vi "NI-USB6343.vi"() -> ()   [LabVIEW 2020]
uses:
  LabVIEW 2020 Toolkits/VI Server Toolkit/VI Server Toolkit LV2013.lvlib
  LabVIEW 2020 Toolkits/toolkits_lv2020_32bit/Synchronization.llb/SynchRefs_SetGet.ctl
  LabVIEW 2020 Toolkits/VI Server Toolkit/VI Server Libraries/VI Server_GetControl.llb/VI Server_STR_Get.vi
  LabVIEW 2020 Toolkits/VI Server Toolkit/VI Server Libraries/VI Server_Set Controls.llb/Set STR Control.vi
  LabVIEW 2020 Toolkits/VI Server Toolkit/VI Server Libraries/VI Server_GetControl.llb/VI Server_DAQmx_Device_Get.vi
panel:
  in  "LastAction.AddToSecuence":bool
  out "System.Message":string caption="System Message"
  in  "Help":bool
  in  "FP.Hide":bool caption="FrontPanel.Hide"
  in  "EXIT":bool
  in  "Tab.Main":T1(tab)
  out "AI.ActualSampleRate":dbl=1000.0 caption="Actual Sample Rate" format="%0.2f"
  out "AI.WaveformGraph":waveform(dbl)(graph) caption="Waveform Graph"
  out "AI.Averaged.Mesurement":dbl caption="Averaged Mesurement" format="%0.4f V"
  in  "AI.Measure":bool caption="AI:Measure"
  in  "AI.Number.Of.Samples":i32=100 caption="Number Of Samples"
  in  "AI.SampleRate":dbl=1000.0 caption="Sample Rate" format="%0.0f Hz"
  in  "AI.MinInputLimit":dbl caption="Min Input Limit" min=-10.0 max=10.0 format="%0.3f V"
  in  "AI.MaxInputLimit":dbl caption="Max Input Limit" min=-10.0 max=10.0 format="%0.3f V"
  in  "AI.TerminalConfiguration":u16(ring)=65535 caption="Terminal Configuration" items=["default"=65535, "RSE"=10083, "NRSE"=10078, "Differential"=10106, "Pseudodifferential"=12529]
  in  "AI.Sample.Mode":u16(ring)=12522 caption="Sample Mode" items=["Finite Samples"=10178, "Continuous Samples"=10123]
  in  "AI.Physical.Channel":tag="Dev1/ai0" caption="Physical Channel"
  in  "AO.GenerationMode":u16(ring) caption="Generation Mode" items=["Voltage DC", "Voltage Sine Wave Generation", "Voltage Triangle Wave Generation", "Voltage Square Wave Generation", "Voltage Sawtooth Wave Generation"]
  in  "AO.Physical.Channel":tag="Dev1/ai0" caption="Physical Channel"
  in  "AO.Update":bool
  in  "AO.Output":bool caption="AO:Output"
  out "AO.WaveformGraph":waveform(dbl)(graph) caption="Waveform Graph"
  in  "AO.SampleMode":u16(ring) caption="Sample Mode" items=["Finite Samples"=10178, "Continious Samples"=10123, "Hardware Timed Single Point"=12522]
  in  "AO.NumberOfSamples":i32=1000 caption="Number Of Samples" min=2
  in  "AO.SampleRate":dbl=1000.0 caption="Sample Rate" format="%0.1f Hz"
  in  "AO.Sample.Clock.Source":tag="OnboardClock" caption="Sample Clock Source"
  out "AO.ActualSampleRate":dbl=1000.0 caption="Actual Sample Rate" format="%0.2f"
  in  "AO.OutputVoltage":dbl(slide) caption="Amplitude" min=-10.0 max=10.0 scale=-10.0..9.0 scale format="%0.3f V"
  in  "AO.SinewaveFrequency":dbl=10.0 caption="Sinewave Frequency" format="%0.2p Hz"
  in  "AO.MaxVoltage":dbl=5.0 caption="Max Voltage" format="%0.3f V"
  in  "AO.MinVoltage":dbl=-5.0 caption="Min Voltage" format="%0.3f V"
  in  "DO.Port.Mask.Apply":bool caption="DO:Port.Mask.Apply"
  in  "DO.Port.Lines.31:24.Mask":u8 caption="Port&Lines 31:24" format="%08b"
  in  "DO.Port.Lines.23:16.Mask":u8 caption="Port&Lines 23:16" format="%08b"
  in  "DO.Port.Lines.15:8.Mask":u8 caption="Port&Lines 15:8" format="%08b"
  in  "DO.Port.Lines.7:0.Mask":u8 caption="Port&Lines 7:0" format="%08b"
  out "DO.Port.State.Verify":bool caption="Verified"
  out "DO.Line.State.Verify":bool caption="Verified"
  in  "DO.Line.State":bool caption="State"
  in  "DO.Line":tag="Dev1/port0/line0:7" caption="Line"
  in  "DO.Line.Update":bool caption="Update:"
  in  "DO.Port.Update":bool caption="DO:Port.Update"
  in  "DO.Port.Lines.31:24":u8 caption="Port&Lines 31:24" format="%08b"
  in  "DO.Port.Lines.23:16":u8 caption="Port&Lines 23:16" format="%08b"
  in  "DO.Port.Lines.15:8":u8 caption="Port&Lines 15:8" format="%08b"
  in  "DO.Port.Lines.7:0":u8 caption="Port&Lines 7:0" format="%08b"
  in  "DO.Port":tag="Dev1/port0/line0:7" caption="Port"
  out "DI.Line.State":bool caption="State"
  in  "DI.Port.Update":bool caption="DI:Port.Update"
  out "DI.Port.Lines.24:31":u8 caption="Port&Lines 31:24" format="%08b"
  out "DI.Port.Lines.16:23":u8 caption="Port&Lines 23:16" format="%08b"
  out "DI.Port.Lines.8:15":u8 caption="Port&Lines 15:8" format="%.0b"
  out "DI.Port.Lines.0:7":u8 caption="Port&Lines 7:0" format="%.0b"
  in  "DI.Port":tag="Dev1/port0/line0:7" caption="Port"
  in  "DI.Line":tag="Dev1/port0/line0:7" caption="Line"
  in  "DI.Line.Update":bool caption="Update:"
  out "ctr3.Out.Duty Cycle.Actual":dbl caption="Ctr3: Duty Cycle Actual" format="%.2f"
  out "ctr3.Out.Frequency.Actual":dbl caption="Ctr3: Frequency Actual" format="%0.3f Hz"
  out "ctr2.Out.Duty Cycle.Actual":dbl caption="Ctr2: Duty Cycle Actual" format="%.2f"
  out "ctr2.Out.Frequency.Actual":dbl caption="Ctr2: Frequency Actual" format="%0.3f Hz"
  out "ctr1.Out.Duty Cycle.Actual":dbl caption="Ctr1: Duty Cycle Actual" format="%.2f"
  out "ctr1.Out.Frequency.Actual":dbl caption="Ctr1: Frequency Actual" format="%0.3f Hz"
  out "ctr0.Out.Duty Cycle.Actual":dbl caption="Ctr0: Duty Cycle Actual" format="%.2f"
  out "ctr0.Out.Frequency.Actual":dbl caption="Ctr0: Frequency Actual" format="%0.3f Hz"
  in  "Cntr.Out.NumberOfPulses":i32=1000 caption="Number Of Pulses" min=1
  in  "Cntr.Out.Start":bool
  in  "Cntr.Out.Sample.Mode":u16(ring)=10123 caption="Sample Mode" items=["Finite Samples"=10178, "Continuous Samples"=10123, "Hardware Timed Single Point"=12522]
  in  "Cntr.Out.Duty.Cycle":dbl=0.5 caption="Duty Cycle" format="%.2f %"
  in  "Cntr.Out.Frequency":dbl=1.0 caption="Frequency" format="%0.3f Hz"
  in  "Cntr.Out.Output.Terminal":tag="/Dev1/PFI12" caption="Output Terminal"
  in  "Cntr.Out.Channel":tag="Dev1/ctr0" caption="Channel"
  out "ctr3.In.Count":u32 caption="Count.3:"
  out "ctr2.In.Count":u32 caption="Count.2:"
  out "ctr1.In.Count":u32 caption="Count.1:"
  out "ctr0.In.Count":u32 caption="Count.0:"
  in  "Cntr.In.Start":bool
  in  "Cntr.In.IntegrationTime":u32=10 format="%.0f msec"
  in  "Cntr.In.Sample.Clock.Source":tag="PFI0" caption="Sample Clock Source"
  in  "Cntr.In.ActiveEdge":u16(ring)=10280 caption="Active Edge" items=["Rising"=10280, "Falling"=10171]
  in  "Cntr.In.Input.Terminal":tag="PFI8" caption="Input.Terminal"
  in  "Cntr.In.Channel":tag="Dev1/port0/line0:7" caption="Channel Name"
  in  "TestCase.Execute.All":bool
  in  "TestCase.Execute.Selected":bool
  out "TestCase.SAVE.Success":bool
  in  "TestCase.SAVE":bool
  in  "SequenceFile.Open":bool
  in  "SequenceFile":path caption="Secuence File"
  in  "TestCase.Execute.Step.Pause":bool
  in  "TestCase.Execute.Steps":u16(ring) caption="Test Case: Pause After Step" items=["1", "2", "3", "4"]
  in  "TestCase.Execute.ABORT":bool
  in  "TestCase.Execute.Next":bool
  in  "TestCase.Execute.Pause":bool
  out "TestCase.ExecutionTime":dbl caption="Execution Time:" format="%0.3f sec"
  in  "TestCase.Execution.StepTime":u32 caption="Seq. Execution: Step Time" format="%d msec"
  in  "TestCaseConfiguration":i32[](listbox) caption="Test Case Configuration"
  in  "TestCase.StepDescription":string caption="Step Description:"
  in  "ProductType":string="USB-6343 (BNC)" caption="Product Type"
  in  "VI.WindowsTitle":string caption="Windows Title"
  in  "DAQmx.Device":tag caption="DAQmx: Device"
  in  "Cont.Measurements.CycleTime":u32 caption="Continius Measurements:\nCycleTime"
  in  "UDP.Test.String2.Send":bool
  in  "UDP.Test.String2":string caption="UDP: Test String 2"
  in  "UDP.Port.BC":u16=58433 caption="UDP: Port.BC"
  in  "UDP.Port.RT":u16=58432 caption="UDP: Port.RT"
  in  "UDP.LocalPort":u16=58434 caption="UDP: Local Port"
  in  "UDP.IP.Address":string="234.5.6.7" caption="UDP: IP Address"
  in  "UDP.Test.String1.Send":bool
  in  "UDP.Test.String1":string caption="UDP: Test String 1"
  in  "UDP.Responce.String.Monitor":bool
  out "UDP.ExecEng.Message.String":string caption="UDP: Execution Engine Message String"
  out "error out":errorcluster={"status"=TRUE, "code"=1055, "source"="Property Node in VI Server Toolkit LV2013.lvlib:VI server_Set Control Value from String Format.vi:5200001->DMM6500_UDP_ExecEng_Instruction_APPLY.vi->DMM6500_UDP_MAIN.vi->Keithley2100.vi"}
  in  "error in":errorcluster
  # "Analog Output Configuration (Generic)"
  # "Digital Output Port\nMASK"
  # "Instructions:\n1: Active Bit; 0: Masked Bit"
  # "Digital Output"
  # "Digital Input"
  # "Counter Input"
  # "Counter Input"
  # "Counter Output"
  # "M"
  # "Multicast IP addresses must be in the 224.0.0.0 to 239.255.255.255 range."
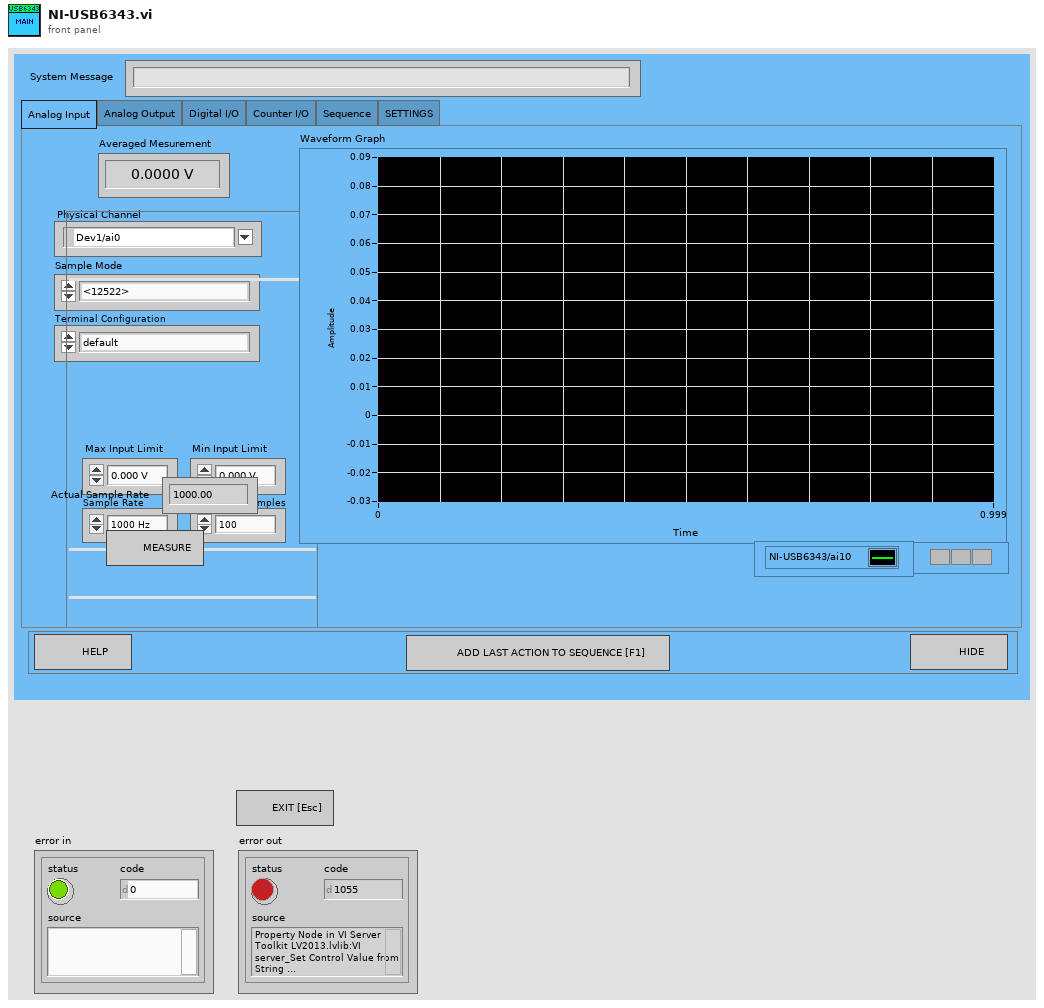
[diagram p1: front panel]
types:
  T1 = enum32{"Analog Input", "Analog Output", "Digital I/O", "Counter I/O", "Sequence", "SETTINGS"}
  T2 = typedef "VI Server_RefsCluster.ctl" = cluster{"Labels":string[], "Refs":refnum<vi>[], "VI Ref":refnum<vi>}
  T3 = typedef "SynchRefs_SetGet.ctl" = enum16{"Set", "Get"}
  T4 = enum8{"Enabled", "Disabled", "Disabled and Grayed Out"}
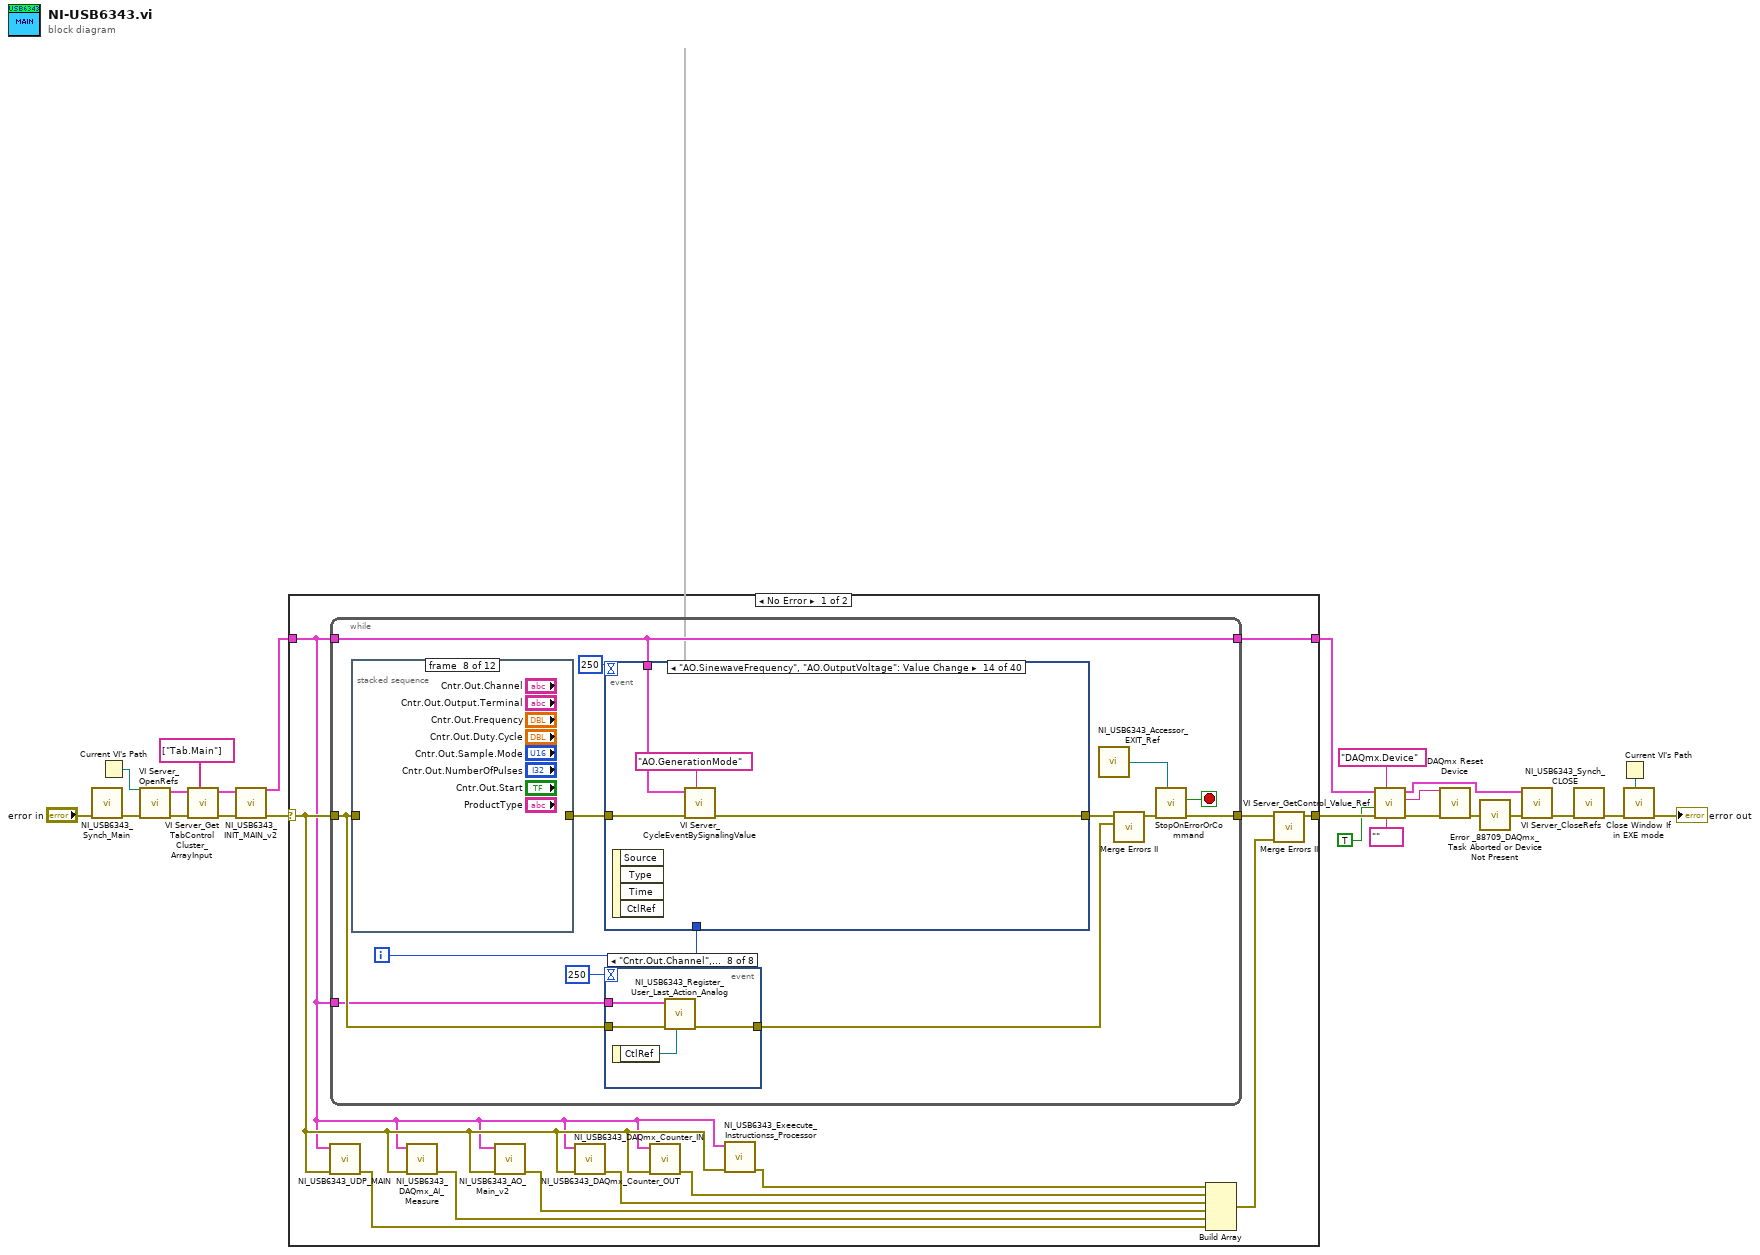
[diagram p0: block diagram]
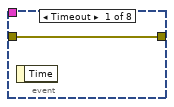
[diagram p2: hidden frame]
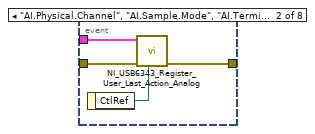
[diagram p3: hidden frame]
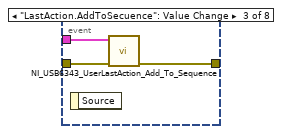
[diagram p4: hidden frame]
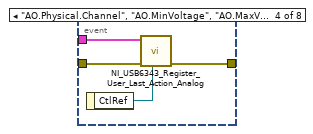
[diagram p5: hidden frame]
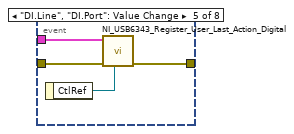
[diagram p6: hidden frame]
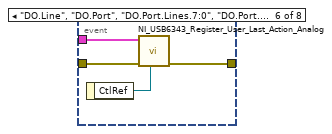
[diagram p7: hidden frame]
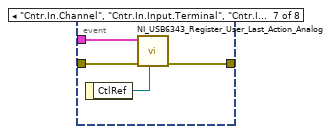
[diagram p8: hidden frame]
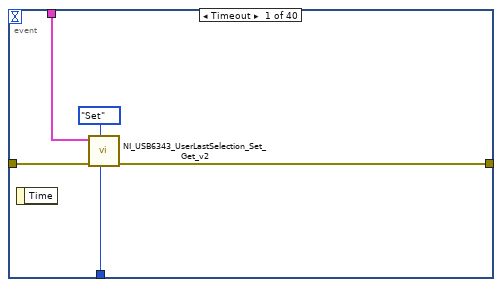
[diagram p9: hidden frame]
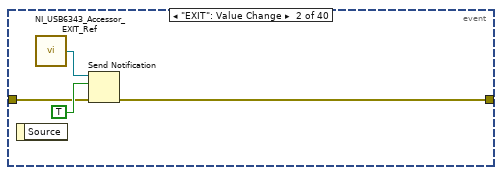
[diagram p10: hidden frame]
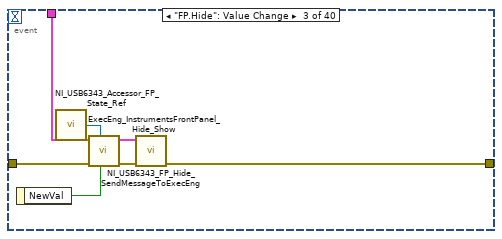
[diagram p11: hidden frame]
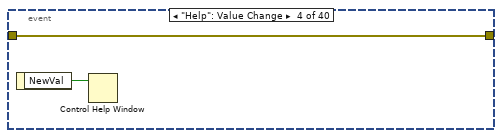
[diagram p12: hidden frame]
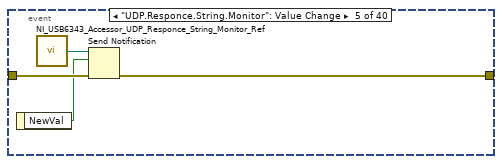
[diagram p13: hidden frame]
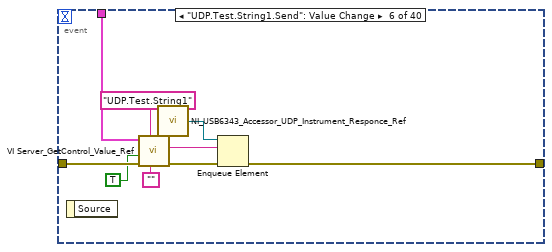
[diagram p14: hidden frame]
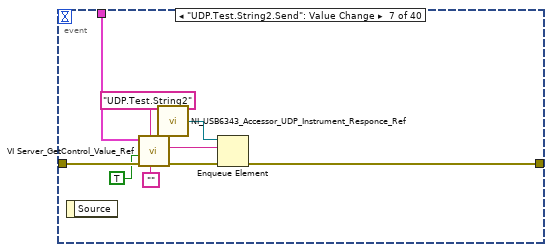
[diagram p15: hidden frame]
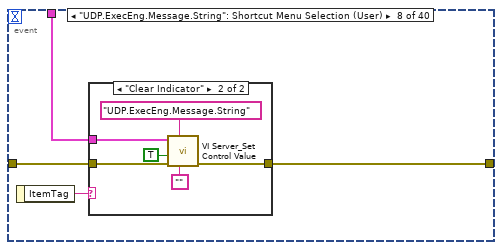
[diagram p16: hidden frame]
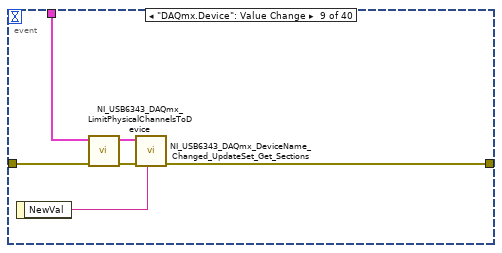
[diagram p18: hidden frame]
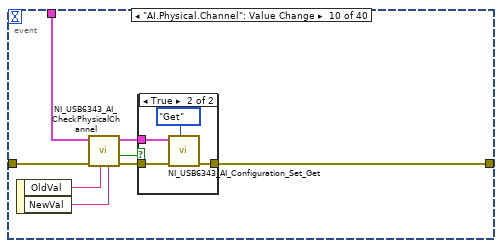
[diagram p19: hidden frame]
diagram:
  n1 = call "NI_USB6343_Synch_Main.vi"("error in"="error in") -> ("error out"=w19:errorcluster)  [unwired: 10 in]
  n2 = Current VI's Path() -> (path=w23:path)
  n3 = call "VI Server_OpenRefs.vi"("error in"=w19, "VI Path"=w23) -> ("error out"=w20:errorcluster, "VI Server.RefsCluster"=w21:T2)  [unwired: 8 in]
  n4 = call "VI Server_Get TabControl Cluster_ArrayInput.vi"("TabControl Labels[]"=string[] ["Tab.Main"], "error in"=w20, "VI Server Cluster"=w21) -> ("error out"=w18:errorcluster, "VI Server Cluster.OUT"=w17:T2)  [unwired: 7 in]
  n5 = call "NI_USB6343_INIT_MAIN_v2.vi"("error in (no error)"=w18, "VI Server Cluster"=w17) -> ("error out"=w16:errorcluster, "VI Server Cluster DUP"=w15:T2)  [unwired: 8 in]
  n6 = case shown="No Error" w16 {
    selector: w16 -> [w27 w298]
    tunnel: [w33 w298] -> w9
    tunnel: w15 -> [w25 w297]
    tunnel: [w36 w297] -> w7
    frame No Error {
      n7 = call "NI_USB6343_UDP_MAIN.vi"("error in (no error)"=w27, "VI Server.RefsCluster"=w25) -> ("error out"=w35:errorcluster)  [unwired: 9 in]
      n8 = while {
        tunnel: w27 -> [w41]
        tunnel: [w45] -> w34
        tunnel: w25 -> [w46]
        tunnel: [w46] -> w36
        tunnel: w25 -> [w37]
        i -> [w47]
        stop <- w44 stop-if-true
        n9 = stacked-sequence {
          tunnel: w41 -> [w296 _ _ _ _ _ _ _ _ _ _ _]
          tunnel: [w296 _ _ _ _ _ _ _ _ _ _ _] -> w49
          frame #0 {
          }
          frame #1 {
          }
          frame #2 {
          }
          frame #3 {
          }
          frame #4 {
          }
          frame #5 {
          }
          frame #6 {
          }
          frame #7 {
          }
          frame #8 {
          }
          frame #9 {
          }
          frame #10 {
          }
          frame #11 {
          }
        }
        n10 = event shown="[13] \"AO.SinewaveFrequency\", \"AO.OutputVoltage\": Value Change" {
          selector: _ -> [_ _ _ _ _ _ _ _ _ _ _ _ _ _ _ _ _ _ _ _ _ _ _ _ _ _ _ _ _ _ _ _ _ _ _ _ _ _ _ _]
          dyn-events: _ -> [_ _ _ _ _ _ _ _ _ _ _ _ _ _ _ _ _ _ _ _ _ _ _ _ _ _ _ _ _ _ _ _ _ _ _ _ _ _ _ _]
          timeout: 250 -> [_ _ _ _ _ _ _ _ _ _ _ _ _ _ _ _ _ _ _ _ _ _ _ _ _ _ _ _ _ _ _ _ _ _ _ _ _ _ _ _]
          tunnel: w49 -> [w81 w83 w93 w95 w99 w108 w117 w121 w134 w140 w148 w152 w159 w163 w167 w174 w181 w193 w197 w200 w203 w207 w210 w213 w222 w230 w233 w238 w249 w255 w258 w261 w265 w268 w269 w274 w278 w287 w291 w295]
          tunnel: w47 -> [w80 _ _ _ _ _ _ _ _ _ _ _ _ _ _ _ _ _ _ _ _ _ _ _ _ _ _ _ _ _ _ _ _ _ _ _ _ _ _ _]
          tunnel: [w78 w85 w87 w95 w97 w106 w115 w119 w131 w142 w148 w149 w153 w160 w164 w169 w179 w192 w195 w198 w201 w206 w208 w211 w219 w228 w234 w236 w243 w254 w256 w260 w263 w267 w270 w272 w276 w282 w290 w292] -> w40
          tunnel: w46 -> [w79 _ w91 _ _ w105 w114 w118 w133 w139 _ w151 w158 w162 _ _ w180 w191 w196 w199 w202 w205 w209 w212 _ w229 w232 w237 w248 w253 w257 w259 w264 w266 w271 w273 _ _ _ _]
          event Timeout {
            n11 = event-data() -> ()  [unwired: 1 in, 1 out]
            n12 = call "NI_USB6343_UserLastSelection_Set_Get_v2.vi"("LoopCounter"=w80, "SynchRefs.Set/Get"=SynchRefs_SetGet."Set", "error in"=w81, "VI Server.RefsCluster"=w79) -> ("error out"=w78:errorcluster)  [unwired: 6 in, 1 out]
          }
          event "EXIT": Value Change {
            n13 = event-data() -> ()  [unwired: 1 in, 1 out]
            n14 = call "NI_USB6343_Accessor_EXIT_Ref.vi"() -> ("EXIT"=w86:refnum<notifier>)  [unwired: 6 in]
            n15 = Send Notification(notification=TRUE, notifier=w86, error in (no error)=w83) -> (error out=w85:errorcluster)  [unwired: 1 out]
          }
          event "FP.Hide": Value Change {
            n16 = event-data() -> ("NewVal"=w92:bool)  [unwired: 1 in]
            n17 = call "NI_USB6343_Accessor_FP_State_Ref.vi"() -> ("FP.State"=w90:refnum<notifier>)  [unwired: 6 in]
            n18 = call "ExecEng_InstrumentsFrontPanel_Hide_Show.vi"("FP.Hide/Show"=w92, "FP.State"=w90, "error in (no error)"=w93, "VI Server Cluster"=w91) -> ("error out"=w88:errorcluster, "VI Server Cluster DUP"=w89:T2)  [unwired: 6 in]
            n19 = call "NI_USB6343_FP_Hide_SendMessageToExecEng.vi"("error in (no error)"=w88, "VI Server Cluster"=w89) -> ("error out"=w87:errorcluster)  [unwired: 9 in]
          }
          event "Help": Value Change {
            n20 = event-data() -> ("NewVal"=w94:bool)  [unwired: 1 in]
            n21 = Control Help Window(1:w94) -> ()  [unwired: 1 in]
          }
          event "UDP.Responce.String.Monitor": Value Change {
            n22 = event-data() -> ("NewVal"=w96:bool)  [unwired: 1 in]
            n23 = call "NI_USB6343_Accessor_UDP_Responce_String_Monitor_Ref.vi"() -> ("UDP.ExecEng.Command.String.Monitor"=w98:refnum<notifier>)  [unwired: 6 in]
            n24 = Send Notification(notification=w96, notifier=w98, error in (no error)=w99) -> (error out=w97:errorcluster)  [unwired: 1 out]
          }
          event "UDP.Test.String1.Send": Value Change {
            n25 = event-data() -> ()  [unwired: 1 in, 1 out]
            n26 = call-poly "VI Server_GetControl_Value_Ref.vi"("DataType"="", "Control.Label"="UDP.Test.String1", "error in"=w108, "SingleInstance"=TRUE, "VI Server.RefsCluster"=w105) -> ("error out"=w107:errorcluster, "Value"=w100:string)  [unwired: 3 in, 2 out]
            n27 = call "NI_USB6343_Accessor_UDP_Instrument_Responce_Ref.vi"() -> ("UDP.Instrument.Responce.Q"=w101:refnum<queue>)  [unwired: 6 in]
            n28 = Enqueue Element(queue=w101, element=w100, error in (no error)=w107) -> (error out=w106:errorcluster)  [unwired: 1 in, 2 out]
          }
          event "UDP.Test.String2.Send": Value Change {
            n29 = event-data() -> ()  [unwired: 1 in, 1 out]
            n30 = call-poly "VI Server_GetControl_Value_Ref.vi"("DataType"="", "Control.Label"="UDP.Test.String2", "error in"=w117, "SingleInstance"=TRUE, "VI Server.RefsCluster"=w114) -> ("error out"=w116:errorcluster, "Value"=w109:string)  [unwired: 3 in, 2 out]
            n31 = call "NI_USB6343_Accessor_UDP_Instrument_Responce_Ref.vi"() -> ("UDP.Instrument.Responce.Q"=w110:refnum<queue>)  [unwired: 6 in]
            n32 = Enqueue Element(queue=w110, element=w109, error in (no error)=w116) -> (error out=w115:errorcluster)  [unwired: 1 in, 2 out]
          }
          event "UDP.ExecEng.Message.String": Shortcut Menu Selection (User) {
            n33 = event-data() -> ("ItemTag"=w120:string)  [unwired: 1 in]
            n34 = case shown="\"Clear Indicator\"" w120 {
              tunnel: w121 -> [w122 w128]
              tunnel: [w122 w127] -> w119
              tunnel: w118 -> [_ w126]
              frame "", Default {
              }
              frame "Clear Indicator" {
                n35 = call-poly "VI Server_Set Control Value.vi"("New Value"="", "Label"="UDP.ExecEng.Message.String" ("Control.Label"), "error in"=w128, "Single Instance (T)"=TRUE ("SingleInstance"), "VI Server Cluster"=w126) -> ("error out"=w127:errorcluster)  [unwired: 4 in, 2 out]
              }
            }
          }
          event "DAQmx.Device": Value Change {
            n36 = event-data() -> ("NewVal"=w129:tag)  [unwired: 1 in]
            n37 = call "NI_USB6343_DAQmx_LimitPhysicalChannelsToDevice.vi"("error in (no error)"=w134, "VI Server Cluster"=w133) -> ("error out"=w132:errorcluster, "VI Server Cluster.DUP"=w130:T2)  [unwired: 7 in, 1 out]
            n38 = call "NI_USB6343_DAQmx_DeviceName_Changed_UpdateSet_Get_Sections.vi"("DAQmx.Device"=w129, "error in (no error)"=w132, "VI Server Cluster"=w130) -> ("error out"=w131:errorcluster)  [unwired: 8 in]
          }
          event "AI.Physical.Channel": Value Change {
            n39 = event-data() -> ("OldVal"=w137:tag, "NewVal"=w136:tag)  [unwired: 1 in]
            n40 = call "NI_USB6343_AI_CheckPhysicalChannel.vi"("NewVal"=w136, "OldVal"=w137, "error in (no error)"=w140, "VI Server Cluster"=w139) -> ("error out"=w141:errorcluster, "AI.Settings.Update"=w135:bool, "VI Server Cluster DUP"=w138:T2)  [unwired: 5 in]
            n41 = case shown="True" w135 {
              tunnel: [w143 w146] -> w142
              tunnel: w141 -> [w143 w145]
              tunnel: w138 -> [_ w144]
              frame False {
              }
              frame True {
                n42 = call "NI_USB6343_AI_Configuration_Set_Get.vi"("SynchRefs.Set/Get"=SynchRefs_SetGet."Get", "error in (no error)"=w145, "VI Server Cluster"=w144) -> ("error out"=w146:errorcluster)  [unwired: 6 in, 2 out]
              }
            }
          }
          event "AI.Measure": Value Change {
            n43 = event-data() -> ()  [unwired: 1 in, 1 out]
          }
          event "AO.Physical.Channel": Value Change {
            n44 = event-data() -> ()  [unwired: 1 in, 1 out]
            n45 = call "NI_USB6343_AO_Configuration_Set_Get.vi"("SynchRefs.Set/Get"=SynchRefs_SetGet."Get", "error in (no error)"=w152, "VI Server Cluster"=w151) -> ("error out"=w149:errorcluster)  [unwired: 6 in, 2 out]
          }
          event "AO.GenerationMode": Value Change {
            n46 = event-data() -> ("NewVal"=w157:u16)  [unwired: 1 in]
            n47 = call "NI_USB6343_AO_GenerationMode.vi"("AO.GenerationMode"=w157, "error in (no error)"=w159, "VI Server Cluster"=w158) -> ("error out"=w154:errorcluster)  [unwired: 7 in, 1 out]
            n48 = call "NI_USB6343_Accessor_ao_Waveform_Array_Update_Ref.vi"() -> ("ao.Waveform.Array.Update"=w156:refnum<notifier>)  [unwired: 6 in]
            n49 = Send Notification(notification=TRUE, notifier=w156, error in (no error)=w154) -> (error out=w153:errorcluster)  [unwired: 1 out]
          }
          event "AO.SinewaveFrequency", "AO.OutputVoltage": Value Change {
            n50 = event-data() -> ()  [unwired: 1 in, 4 out]
            n51 = call "VI Server_CycleEventBySignalingValue.vi"("Label"="AO.GenerationMode", "error in"=w163, "VI Server.RefsCluster"=w162) -> ("error out"=w160:errorcluster)  [unwired: 7 in, 1 out]
          }
          event "AO.Update": Value Change {
            n52 = event-data() -> ()  [unwired: 1 in, 1 out]
            n53 = call "NI_USB6343_Accessor_ao_Waveform_Array_Update_Ref.vi"() -> ("ao.Waveform.Array.Update"=w166:refnum<notifier>)  [unwired: 6 in]
            n54 = Send Notification(notification=TRUE, notifier=w166, error in (no error)=w167) -> (error out=w164:errorcluster)  [unwired: 1 out]
          }
          event "AO.Output": Value Change {
            n55 = event-data() -> ("NewVal"=w172:bool)  [unwired: 1 in]
            n56 = call "NI_USB6343_Accessor_ao0_State_Ref.vi"() -> ("ao0.State"=w173:refnum<notifier>)  [unwired: 6 in]
            n57 = Send Notification(notification=w172, notifier=w173, error in (no error)=w174) -> (error out=w170:errorcluster)  [unwired: 1 out]
            n58 = call "NI_USB6343_Accessor_ao_Waveform_Array_Update_Ref.vi"() -> ("ao.Waveform.Array.Update"=w171:refnum<notifier>)  [unwired: 6 in]
            n59 = Send Notification(notification=TRUE, notifier=w171, error in (no error)=w170) -> (error out=w169:errorcluster)  [unwired: 1 out]
          }
          event "AO.Sample.Clock.Source", "AO.SampleMode", "AO.SampleRate", "AO.NumberOfSamples", "AO.MaxVoltage", "AO.MinVoltage": Value Change {
            n60 = event-data() -> ()  [unwired: 1 in, 1 out]
            n61 = call "NI_USB6343_AO_ConfigurationAtributes.vi"("error in (no error)"=w181, "VI Server Cluster"=w180) -> ("error out"=w178:errorcluster)  [unwired: 8 in, 1 out]
            n62 = call "NI_USB6343_Accessor_ao0_State_Ref.vi"() -> ("ao0.State"=w176:refnum<notifier>)  [unwired: 6 in]
            n63 = Get Notifier Status(notifier=w176, error in (no error)=w178) -> (current notification=w175:bool, error out=w177:errorcluster)  [unwired: 3 out]
            n64 = case shown="True" w175 {
              tunnel: [w182 w187] -> w179
              tunnel: w177 -> [w182 w184]
              tunnel: w176 -> [_ w183]
              frame False {
              }
              frame True {
                w186 = TRUE ("notification")
                n65 = Send Notification(notification=FALSE, notifier=w183, error in (no error)=w184) -> (error out=w189:errorcluster)  [unwired: 1 out]
                n66 = call "NI_USB6343_Accessor_ao_Waveform_Array_Update_Ref.vi"() -> ("ao.Waveform.Array.Update"=w190:refnum<notifier>)  [unwired: 6 in]
                n67 = Send Notification(notification=w186, notifier=w190, error in (no error)=w189) -> (error out=w188:errorcluster)  [unwired: 1 out]
                n68 = Send Notification(notification=w186, notifier=w183, error in (no error)=w188) -> (error out=w187:errorcluster)  [unwired: 1 out]
              }
            }
          }
          event "DI.Line.Update": Value Change {
            n69 = event-data() -> ()  [unwired: 1 in, 1 out]
            n70 = call "NI_USB6343_Digital_Input_Line_Update.vi"("error in (no error)"=w193, "VI Server Cluster"=w191) -> ("error out"=w192:errorcluster)  [unwired: 9 in]
          }
          event "DI.Port": Value Change {
            n71 = event-data() -> ("NewVal"=w194:tag)  [unwired: 1 in]
            n72 = call "NI_USB6343_DI_Port_ValueChanged.vi"("DI.Port"=w194, "error in (no error)"=w197, "VI Server Cluster"=w196) -> ("error out"=w195:errorcluster)  [unwired: 8 in]
          }
          event "DI.Port.Update": Value Change {
            n73 = event-data() -> ()  [unwired: 1 in, 1 out]
            n74 = call "NI_USB6343_DI_Port_Update.vi"("error in (no error)"=w200, "VI Server Cluster"=w199) -> ("error out"=w198:errorcluster)  [unwired: 9 in]
          }
          event "DO.Line.Update": Value Change {
            n75 = event-data() -> ()  [unwired: 1 in, 1 out]
            n76 = call "NI_USB6343_Digital_Output_Line_Update.vi"("error in (no error)"=w203, "VI Server Cluster"=w202) -> ("error out"=w201:errorcluster)  [unwired: 9 in]
          }
          event "DO.Port": Value Change {
            n77 = event-data() -> ("NewVal"=w204:tag)  [unwired: 1 in]
            n78 = call "NI_USB6343_DO_Port_ValueChanged.vi"("DO.Port"=w204, "error in (no error)"=w207, "VI Server Cluster"=w205) -> ("error out"=w206:errorcluster)  [unwired: 8 in]
          }
          event "DO.Port.Update": Value Change {
            n79 = event-data() -> ()  [unwired: 1 in, 1 out]
            n80 = call "NI_USB6343_DO_Port_Update.vi"("error in (no error)"=w210, "VI Server Cluster"=w209) -> ("error out"=w208:errorcluster)  [unwired: 9 in]
          }
          event "DO.Port.Mask.Apply": Value Change {
            n81 = event-data() -> ()  [unwired: 1 in, 1 out]
            n82 = call "NI_USB6343_DO_Port_Mask_Apply.vi"("error in (no error)"=w213, "VI Server Cluster"=w212) -> ("error out"=w211:errorcluster)  [unwired: 9 in]
          }
          event "DO.Port.Lines.7:0", "DO.Port.Lines.15:8", "DO.Port.Lines.23:16", "DO.Port.Lines.31:24", "DO.Port.Lines.7:0.Mask", "DO.Port.Lines.15:8.Mask", "DO.Port.Lines.23:16.Mask", "DO.Port.Lines.31:24.Mask", "DI.Port.Lines.0:7", "DI.Port.Lines.8:15", "DI.Port.Lines.16:23", "DI.Port.Lines.24:31": Mouse Down {
            n83 = event-data() -> ("CtlRef"=w221:refnum<vi>)  [unwired: 1 in]
            n84 = property class="DigNum (strict)"(reference=w221, error in=w222) -> (reference out=w218:refnum<vi>, error out=w220:errorcluster, "FormatString"=w215:string)
            n85 = Match Pattern(string=w215, regular expression="[0-9]+") -> (after substring=w214:string)  [unwired: 1 in, 3 out]
            n86 = case shown="\"b\", Default" w214 {
              tunnel: ["%.0f" "%02x" "%02o" "%08b"] -> w217
              frame "f" {
              }
              frame "x" {
              }
              frame "o" {
              }
              frame "b", Default {
              }
            }
            n87 = property class="DigNum (strict)"(reference=w218, error in=w220, "FormatString"=w217) -> (error out=w219:errorcluster)  [unwired: 1 out]
          }
          event "Cntr.In.Channel": Value Change {
            n88 = event-data() -> ("NewVal"=w227:tag)  [unwired: 1 in]
            n89 = call "NI-USB6343_Counter_IN_GetStateFromFile.vi"("Counter.IN.Channel"=w227, "error in (no error)"=w230, "VI Server Cluster"=w229) -> ("error out"=w228:errorcluster)  [unwired: 7 in, 1 out]
          }
          event "Cntr.In.Start": Value Change {
            n90 = event-data() -> ("NewVal"=w231:bool)  [unwired: 1 in]
            n91 = call "NI-USB6343_Counter_IN_SaveStateToFile.vi"("Cntr.In.Start"=w231, "error in (no error)"=w233, "VI Server Cluster"=w232) -> ("error out"=w234:errorcluster)  [unwired: 7 in, 1 out]
          }
          event "Cntr.Out.Channel": Value Change {
            n92 = event-data() -> ("NewVal"=w239:tag, "OldVal"=w235:tag)  [unwired: 1 in]
            n93 = call "NI-USB6343_Counter_OUT_GetStateFromFile.vi"("Counter.OUT.Channel.Old"=w235, "Counter.OUT.Channel.New"=w239, "error in (no error)"=w238, "VI Server Cluster"=w237) -> ("error out"=w236:errorcluster)  [unwired: 6 in, 1 out]
          }
          event "Cntr.Out.Sample.Mode": Value Change {
            n94 = event-data() -> ()  [unwired: 1 in, 1 out]
            n95 = call "VI Server_Get Text Ring Selection.vi"("Label"="Cntr.Out.Sample.Mode", "error in"=w249, "Single Instance (T)"=TRUE, "VI Server Cluster"=w248) -> ("error out"=w244:errorcluster, "Selection"=w245:string, "VI Server Custer.DUP"=w242:T2)  [unwired: 2 in, 3 out]
            n96 = case shown="\"Finite Samples\"" w245 {
              tunnel: [T4."Disabled and Grayed Out" ("Disabled") T4."Enabled" ("Disabled")] -> w241
              frame "Continuous Samples", Default {
              }
              frame "Finite Samples" {
              }
            }
            n97 = call "VI Server_Enable_Disable.vi"("Disabled"=w241, "Label"="Cntr.Out.NumberOfPulses", "error in"=w244, "VI Server Cluster"=w242) -> ("error out"=w243:errorcluster)  [unwired: 5 in, 2 out]
          }
          event "Cntr.Out.Start": Value Change {
            n98 = event-data() -> ("NewVal"=w252:bool)  [unwired: 1 in]
            n99 = call "NI-USB6343_Counter_OUT_SaveStateToFile.vi"("Cntr.In.Start"=w252, "error in (no error)"=w255, "VI Server Cluster"=w253) -> ("error out"=w254:errorcluster)  [unwired: 7 in, 1 out]
          }
          event "TestCase.SAVE": Value Change {
            n100 = event-data() -> ()  [unwired: 1 in, 1 out]
            n101 = call "NI_USB6343_Sequence_Save.vi"("error in (no error)"=w258, "VI Server Cluster"=w257) -> ("error out"=w256:errorcluster)  [unwired: 9 in]
          }
          event "SequenceFile.Open": Value Change {
            n102 = event-data() -> ()  [unwired: 1 in, 1 out]
            n103 = call "NI_USB6343_Sequence_Open.vi"("error in (no error)"=w261, "VI Server Cluster"=w259) -> ("error out"=w260:errorcluster)  [unwired: 9 in]
          }
          event "TestCaseConfiguration": Shortcut Menu Selection (User) {
            n104 = event-data() -> ("ItemTag"=w262:string)  [unwired: 1 in]
            n105 = call "NI_USB6343_Sequence_TestCaseConfig_UserMenu.vi"("ItemTag"=w262, "error in (no error)"=w265, "VI Server.RefsCluster"=w264) -> ("error out"=w263:errorcluster)  [unwired: 8 in]
          }
          event "TestCaseConfiguration": Value Change {
            n106 = event-data() -> ()  [unwired: 1 in, 1 out]
            n107 = call "NI_USB6343_TestCase_Configuration_ValueChanged.vi"("error in"=w268, "VI Server.RefsCluster"=w266) -> ("error out"=w267:errorcluster)  [unwired: 8 in, 1 out]
          }
          event "TestCase.Execute.Selected": Value Change {
            n108 = event-data() -> ()  [unwired: 1 in, 1 out]
            n109 = call "NI_USB6343_ExecuteSelectedInstruction.vi"("error in (no error)"=w269, "VI Server Cluster"=w271) -> ("error out"=w270:errorcluster)  [unwired: 9 in]
          }
          event "TestCase.Execute.All": Value Change {
            n110 = event-data() -> ()  [unwired: 1 in, 1 out]
            n111 = call "NI_USB6343_Execute_All_Instruction.vi"("error in (no error)"=w274, "VI Server Cluster"=w273) -> ("error out"=w272:errorcluster)  [unwired: 9 in]
          }
          event "TestCase.Execute.Pause": Value Change {
            n112 = event-data() -> ("NewVal"=w275:bool)  [unwired: 1 in]
            n113 = call "NI_USB6343_Accessor_Sequence_Execution_Pause_Ref.vi"() -> ("SequenceExecution.PAUSE"=w277:refnum<notifier>)  [unwired: 6 in]
            n114 = Send Notification(notification=w275, notifier=w277, error in (no error)=w278) -> (error out=w276:errorcluster)  [unwired: 1 out]
          }
          event "TestCase.Execute.Next": Value Change {
            n115 = event-data() -> ()  [unwired: 1 in, 1 out]
            n116 = call "NI_USB6343_Accessor_Sequence_Execution_Pause_Ref.vi"() -> ("SequenceExecution.PAUSE"=w281:refnum<notifier>)  [unwired: 6 in]
            n117 = Send Notification(notification=FALSE, notifier=w281, error in (no error)=w287) -> (notifier out=w279:refnum<notifier>, error out=w285:errorcluster)
            n118 = call "Time Delay"("error in (no error)"=w285, "Delay Time (s)"=0.05) -> ("error out"=w283:errorcluster)  [unwired: 9 in]
            n119 = Send Notification(notification=TRUE, notifier=w279, error in (no error)=w283) -> (error out=w282:errorcluster)  [unwired: 1 out]
          }
          event "TestCase.Execute.ABORT": Value Change {
            n120 = event-data() -> ()  [unwired: 1 in, 1 out]
            n121 = call "NI_USB6343_Accessor_Sequence_Execution_ABORT_Ref.vi"() -> ("SequenceExecution.ABORT"=w289:refnum<notifier>)  [unwired: 6 in]
            n122 = Send Notification(notification=TRUE, notifier=w289, error in (no error)=w291) -> (error out=w290:errorcluster)  [unwired: 1 out]
          }
          event "TestCase.Execute.Step.Pause": Value Change {
            n123 = event-data() -> ("NewVal"=w293:bool)  [unwired: 1 in]
            n124 = call "NI_USB6343_TestCase_Execution_Pause_Ref.vi"() -> ("SequenceExecution.StepPAUSE"=w294:refnum<notifier>)  [unwired: 6 in]
            n125 = Send Notification(notification=w293, notifier=w294, error in (no error)=w295) -> (error out=w292:errorcluster)  [unwired: 1 out]
          }
        }
        n126 = event shown="[7] \"Cntr.Out.Channel\", \"Cntr.Out.Output.Terminal\", \"Cntr.Out.Frequency\", \"Cntr.Out.Duty.Cycle\", \"Cntr.Out.Sample.Mode\", \"Cntr.Out.NumberOfPulses\": Value Change" {
          selector: _ -> [_ _ _ _ _ _ _ _]
          dyn-events: _ -> [_ _ _ _ _ _ _ _]
          timeout: 250 -> [_ _ _ _ _ _ _ _]
          tunnel: w41 -> [w50 w54 w57 w61 w65 w69 w73 w77]
          tunnel: [w50 w53 w56 w59 w63 w68 w72 w76] -> w38
          tunnel: w37 -> [_ w51 w55 w60 w64 w66 w70 w74]
          event Timeout {
            n127 = event-data() -> ()  [unwired: 1 in, 1 out]
          }
          event "AI.Physical.Channel", "AI.Sample.Mode", "AI.TerminalConfiguration", "AI.MaxInputLimit", "AI.MinInputLimit", "AI.SampleRate", "AI.Number.Of.Samples": Value Change {
            n128 = event-data() -> ("CtlRef"=w52:refnum<vi>)  [unwired: 1 in]
            n129 = call "NI_USB6343_Register_User_Last_Action_Analog.vi"("Control in"=w52, "error in (no error)"=w54, "VI Server Cluster"=w51) -> ("error out"=w53:errorcluster)  [unwired: 8 in]
          }
          event "LastAction.AddToSecuence": Value Change {
            n130 = event-data() -> ()  [unwired: 1 in, 1 out]
            n131 = call "NI_USB6343_UserLastAction_Add_To_Sequence.vi"("error in (no error)"=w57, "VI Server Cluster"=w55) -> ("error out"=w56:errorcluster)  [unwired: 9 in]
          }
          event "AO.Physical.Channel", "AO.MinVoltage", "AO.MaxVoltage", "AO.Sample.Clock.Source", "AO.SampleRate", "AO.NumberOfSamples", "AO.GenerationMode", "AO.SinewaveFrequency", "AO.SampleMode", "AO.OutputVoltage": Value Change {
            n132 = event-data() -> ("CtlRef"=w58:refnum<vi>)  [unwired: 1 in]
            n133 = call "NI_USB6343_Register_User_Last_Action_Analog.vi"("Control in"=w58, "error in (no error)"=w61, "VI Server Cluster"=w60) -> ("error out"=w59:errorcluster)  [unwired: 8 in]
          }
          event "DI.Line", "DI.Port": Value Change {
            n134 = event-data() -> ("CtlRef"=w62:refnum<vi>)  [unwired: 1 in]
            n135 = call "NI_USB6343_Register_User_Last_Action_Digital.vi"("CtlRef"=w62, "error in (no error)"=w65, "VI Server Cluster"=w64) -> ("error out"=w63:errorcluster)  [unwired: 8 in]
          }
          event "DO.Line", "DO.Port", "DO.Port.Lines.7:0", "DO.Port.Lines.15:8", "DO.Port.Lines.23:16", "DO.Port.Lines.31:24", "DO.Port.Lines.7:0.Mask", "DO.Port.Lines.15:8.Mask", "DO.Port.Lines.23:16.Mask", "DO.Port.Lines.31:24.Mask": Value Change {
            n136 = event-data() -> ("CtlRef"=w67:refnum<vi>)  [unwired: 1 in]
            n137 = call "NI_USB6343_Register_User_Last_Action_Analog.vi"("Control in"=w67, "error in (no error)"=w69, "VI Server Cluster"=w66) -> ("error out"=w68:errorcluster)  [unwired: 8 in]
          }
          event "Cntr.In.Channel", "Cntr.In.Input.Terminal", "Cntr.In.ActiveEdge", "Cntr.In.Sample.Clock.Source", "Cntr.In.IntegrationTime": Value Change {
            n138 = event-data() -> ("CtlRef"=w71:refnum<vi>)  [unwired: 1 in]
            n139 = call "NI_USB6343_Register_User_Last_Action_Analog.vi"("Control in"=w71, "error in (no error)"=w73, "VI Server Cluster"=w70) -> ("error out"=w72:errorcluster)  [unwired: 8 in]
          }
          event "Cntr.Out.Channel", "Cntr.Out.Output.Terminal", "Cntr.Out.Frequency", "Cntr.Out.Duty.Cycle", "Cntr.Out.Sample.Mode", "Cntr.Out.NumberOfPulses": Value Change {
            n140 = event-data() -> ("CtlRef"=w75:refnum<vi>)  [unwired: 1 in]
            n141 = call "NI_USB6343_Register_User_Last_Action_Analog.vi"("Control in"=w75, "error in (no error)"=w77, "VI Server Cluster"=w74) -> ("error out"=w76:errorcluster)  [unwired: 8 in]
          }
        }
        n142 = call "NI_USB6343_Accessor_EXIT_Ref.vi"() -> ("EXIT"=w43:refnum<notifier>)  [unwired: 6 in]
        n143 = call "Merge Errors II.vi"("error in 2 (no error)"=w38, "error in 1 (no error)"=w40) -> ("error out.DUP"=w39:errorcluster)  [unwired: 4 in, 1 out]
        n144 = call "StopOnErrorOrCommand.vi"("STOP"=w43, "error in (no error)"=w39) -> ("error out"=w45:errorcluster, "STOP"=w44:bool)  [unwired: 8 in]
      }
      n145 = call "NI_USB6343_DAQmx_AI_Measure.vi"("error in (no error)"=w27, "VI Server Cluster"=w25) -> ("error out"=w31:errorcluster)  [unwired: 9 in]
      n146 = call "NI_USB6343_AO_Main_v2.vi"("error in (no error)"=w27, "VI Server Cluster"=w25) -> ("error out"=w28:errorcluster)  [unwired: 9 in]
      n147 = call "NI_USB6343_DAQmx_Counter_IN.vi"("error in (no error)"=w27, "VI Server Cluster"=w25) -> ("error out"=w30:errorcluster)  [unwired: 9 in]
      n148 = call "NI_USB6343_DAQmx_Counter_OUT.vi"("error in (no error)"=w27, "VI Server Cluster"=w25) -> ("error out"=w29:errorcluster)  [unwired: 9 in]
      n149 = call "NI_USB6343_Exeecute_Instructionss_Processor.vi"("error in (no error)"=w27, "VI Server.RefsCluster"=w25) -> ("error out"=w26:errorcluster)  [unwired: 9 in]
      n150 = Build Array(w26, w29, w30, w28, w31, w35) -> (w32:errorcluster[])
      n151 = call "Merge Errors II.vi"("error array in"=w32, "error in 1 (no error)"=w34) -> ("error out.DUP"=w33:errorcluster)  [unwired: 4 in, 1 out]
    }
    frame Error {
    }
  }
  n152 = call-poly "VI Server_GetControl_Value_Ref.vi"("DataType"=tag "" ("DAQmx.Device"), "Control.Label"="DAQmx.Device", "error in"=w9, "SingleInstance"=TRUE, "VI Server.RefsCluster"=w7) -> ("error out"=w12:errorcluster, "Value"=w13:tag, "VI Server.RefsCluster.DUP"=w8:T2)  [unwired: 3 in, 1 out]
  n153 = call <vilib>:"DAQmx Reset Device.vi"("device in"=w13, "error in"=w12) -> ("error out"=w2:errorcluster)  [unwired: 13 in]
  n154 = call "Error _88709_DAQmx_Task Aborted or Device Not Present.vi"("error in"=w2) -> ("error out"=w1:errorcluster)  [unwired: 13 in, 1 out]
  n155 = call "VI Server_CloseRefs.vi"("error in"=w1, "VI Server.RefsCluster"=w8) -> ("error out"=w14:errorcluster)  [unwired: 9 in]
  n156 = call "NI_USB6343_Synch_CLOSE.vi"("error in"=w14) -> ("error out"=w5:errorcluster)  [unwired: 10 in]
  n157 = Current VI's Path() -> (path=w3:path)
  n158 = call "Close Window If in EXE mode.vi"("TopLevelVI Path"=w3, "error in"=w5) -> ("error out"=→"error out":errorcluster)  [unwired: 9 in]
